vi "sutter_control.vi"() -> ()   [LabVIEW 2016]
uses:
  <vilib>/Instr/_visa.llb/VISA Configure Serial Port (Instr).vi
panel:
  in  "Driver : 1/2":bool
  in  "error in (no error)":errorcluster
  in  "Go Home":bool
  in  "stop":bool
  out "error out":errorcluster
  out "z-position":dbl
  out "y-position":dbl
  out "x-position":dbl
  in  "Z um":dbl
  in  "Y um":dbl
  in  "X um":dbl
  in  "VISA resource name":refnum<visa-resource-name>
  # "Back to (0 0 0)"
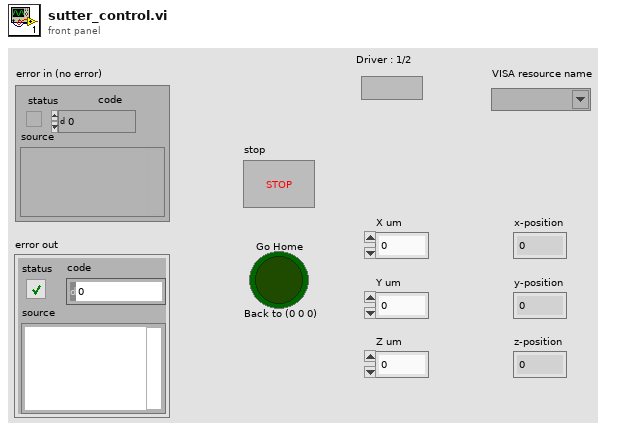
[diagram p1: front panel]
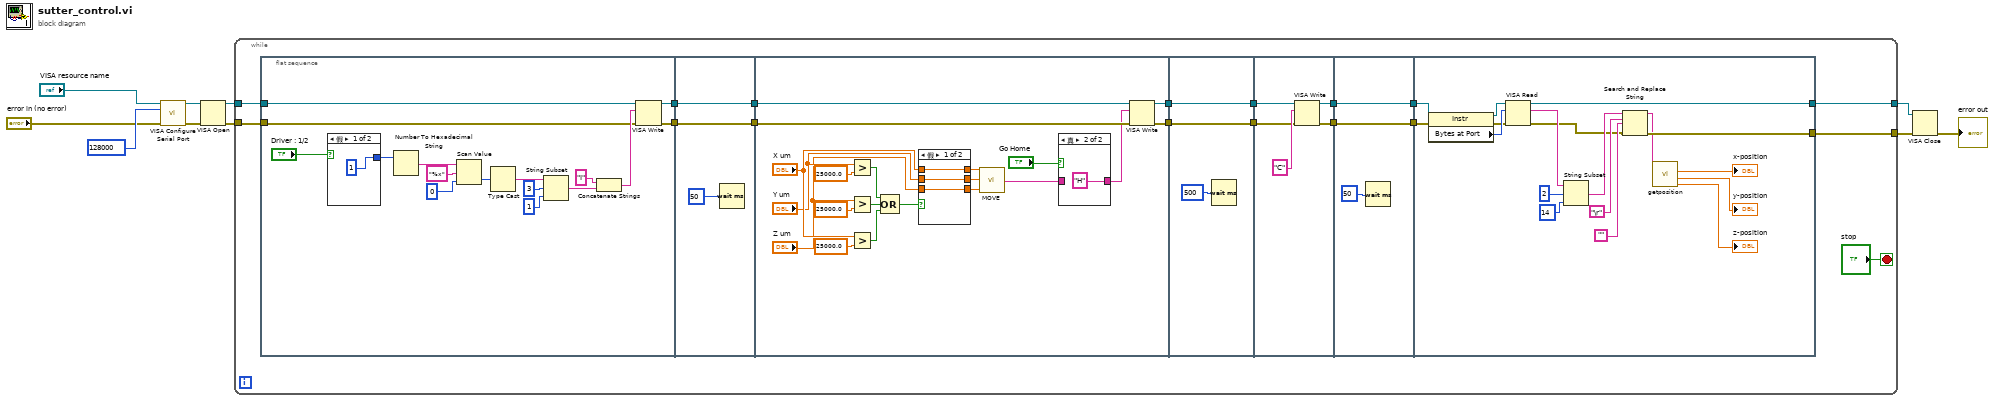
[diagram p0: block diagram]
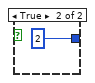
[diagram p2: hidden frame]
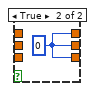
[diagram p4: hidden frame]
diagram:
  n1 = call-poly "VISA Configure Serial Port"("VISA resource name"="VISA resource name", "baud rate (9600)"=u32 128000, "error in (no error)"="error in (no error)") -> ("VISA resource name out"=w6:refnum<visa-resource-name>, "error out"=w2:errorcluster)  [unwired: 11 in]
  n2 = VISA Open(error in (no error)=w2, VISA resource name=w6) -> (VISA resource name=w5:refnum<visa-resource-name>, error out=w1:errorcluster)  [unwired: 3 in]
  n3 = while {
    tunnel: w1 -> [w18]
    tunnel: [w27] -> w7
    tunnel: w5 -> [w25]
    tunnel: [w15] -> w3
    stop <- "stop" stop-if-true
    n4 = flat-sequence {
      tunnel: w18 -> [w29]
      tunnel: w25 -> [w43]
      tunnel: [w31] -> w12
      tunnel: [w28] -> w11
      tunnel: [w48] -> w14
      tunnel: [w47] -> w13
      tunnel: w12 -> [w48]
      tunnel: w11 -> [w47]
      tunnel: [w68] -> w24
      tunnel: [w67] -> w23
      tunnel: w14 -> [w66]
      tunnel: w13 -> [w65]
      tunnel: w24 -> [w77]
      tunnel: [w77] -> w22
      tunnel: [w75] -> w21
      tunnel: w23 -> [w75]
      tunnel: w22 -> [w79]
      tunnel: w21 -> [w81]
      tunnel: [w80] -> w20
      tunnel: [w78] -> w16
      tunnel: w20 -> [w85]
      tunnel: [w85] -> w19
      tunnel: [w83] -> w17
      tunnel: w16 -> [w83]
      tunnel: w19 -> [w98]
      tunnel: [w97] -> w27
      tunnel: w17 -> [w94]
      tunnel: [w92] -> w15
      frame #0 {
        n5 = case shown="假" "Driver : 1/2" {
          tunnel: [1 2] -> w41
          frame False {
          }
          frame True {
          }
        }
        n6 = Number To Hexadecimal String(2:w41) -> (0:w39:string)  [unwired: 1 in]
        n7 = Scan Value(string=w39, format string="%x", default (0 dbl)=0) -> (value=w37:i32)  [unwired: 1 out]
        n8 = Type Cast(x=w37) -> (*(type *) &x=w35:string)  [unwired: 1 in]
        n9 = String Subset(string=w35, offset (0)=3, length (rest)=1 ("length (rest)")) -> (substring=w32:string)
        n10 = Concatenate Strings("I" ("string"), w32) -> (w42:string)
        n11 = VISA Write(VISA resource name=w43, write buffer=w42, error in (no error)=w29) -> (VISA resource name out=w31:refnum<visa-resource-name>, error out=w28:errorcluster)  [unwired: 1 out]
      }
      frame #1 {
        n12 = Wait (ms)(milliseconds to wait=u32 50) -> ()  [unwired: 1 out]
      }
      frame #2 {
        n13 = Greater?(x="Y um", y=25000.0) -> (0:w61:bool)
        n14 = Greater?(x="Z um", y=25000.0) -> (0:w60:bool)
        n15 = Greater?(x="X um", y=25000.0) -> (0:w59:bool)
        n16 = Compound Arithmetic op=OR(w61, w60, w59) -> (w58:bool)
        n17 = case shown="假" w58 {
          tunnel: [w73 w74] -> w57
          tunnel: "X um" -> [w73 _]
          tunnel: [w72 w74] -> w55
          tunnel: "Y um" -> [w72 _]
          tunnel: [w71 w74] -> w53
          tunnel: "Z um" -> [w71 _]
          frame False {
          }
          frame True {
            w74 = 0
          }
        }
        n18 = call "MOVE.vi"("Z"=w53, "Y"=w55, "x"=w57) -> ("MOVE COMMAND"=w49:string)
        n19 = case shown="真" "Go Home" {
          tunnel: [w69 "H" ("MOVE COMMAND")] -> w50
          tunnel: w49 -> [w69 _]
          frame False {
          }
          frame True {
          }
        }
        n20 = VISA Write(VISA resource name=w66, write buffer=w50, error in (no error)=w65) -> (VISA resource name out=w67:refnum<visa-resource-name>, error out=w68:errorcluster)  [unwired: 1 out]
      }
      frame #3 {
        n21 = Wait (ms)(milliseconds to wait=u32 500) -> ()  [unwired: 1 out]
      }
      frame #4 {
        n22 = VISA Write(VISA resource name=w81, write buffer="C", error in (no error)=w79) -> (VISA resource name out=w80:refnum<visa-resource-name>, error out=w78:errorcluster)  [unwired: 1 out]
      }
      frame #5 {
        n23 = Wait (ms)(milliseconds to wait=u32 50) -> ()  [unwired: 1 out]
      }
      frame #6 {
        n24 = property class="Instr"(reference=w98, error in=w94) -> (reference out=w103:refnum<visa-resource-name>, error out=w93:errorcluster, "Bytes at Port"=w99:u32)
        n25 = VISA Read(VISA resource name=w103, byte count=w99, error in (no error)=w93) -> (VISA resource name out=w97:refnum<visa-resource-name>, read buffer=w90:string, error out=w86:errorcluster)  [unwired: 1 out]
        n26 = String Subset(string=w90, offset (0)=2, length (rest)=14 ("length (rest)")) -> (substring=w87:string)
        n27 = Search and Replace String(input string=w87, search string="\r", replace string="", error in=w86) -> (result string=w91:string, error out=w92:errorcluster)  [unwired: 4 in, 2 out]
        n28 = call "getposition.vi"("string"=w91) -> ("x-position"=→"x-position":dbl, "y-position"=→"y-position":dbl, "z-position"=→"z-position":dbl)  [unwired: 1 out]
      }
    }
  }
  n29 = VISA Close(VISA resource name=w7, error in (no error)=w3) -> (error out=→"error out":errorcluster)
